vi "ProbeType.vi"(1 "tcp timeout (ms)":i32=40, 3 "connection ID in":refnum<k5>) -> (0 "ProbeType":i8)   [LabVIEW 2016]
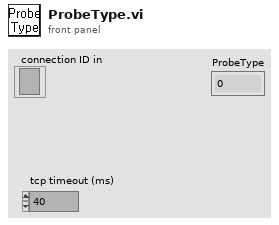
[diagram p1: front panel]
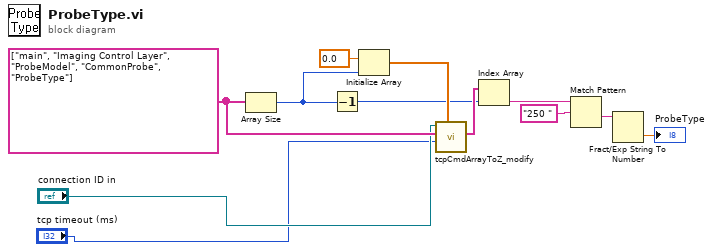
[diagram p0: block diagram]
diagram:
  w10 = string[] ["main", "Imaging Control Layer", "ProbeModel", "CommonProbe", "ProbeType"] ("ScanRange Parameter")
  n1 = Array Size(array=w10) -> (size(s)=w5:i32)
  n2 = Decrement(x=w5) -> (x-1=w4:i32)
  n3 = Initialize Array(sgl 0.0 ("element"), w5) -> (w11:sgl[])
  n4 = call "tcpCmdArrayToZ_modify.vi"("Delay (sec)"=w11, "Timeout (ms)"="tcp timeout (ms)", "Command array"=w10, "connection ID in"="connection ID in") -> ("Receive array"=w6:string[])  [unwired: 3 in, 4 out]
  n5 = Index Array(array=w6, index=w4) -> (element=w8:string)
  n6 = Match Pattern(string=w8, regular expression="250 ") -> (after substring=w7:string)  [unwired: 1 in, 3 out]
  n7 = Fract/Exp String To Number(string=w7) -> (number=→"ProbeType":dbl)  [unwired: 3 in, 1 out]
